vi "get git version.vi"(8 "error in":errorcluster) -> (0 "error out":errorcluster, 2 "hashcode":string, 3 "path to current head":path)   [LabVIEW 2013]
uses:
  <vilib>/regexp/Match Regular Expression.xnode
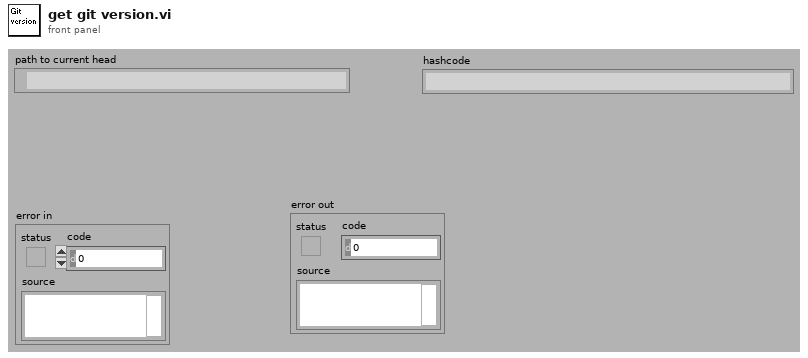
[diagram p1: front panel]
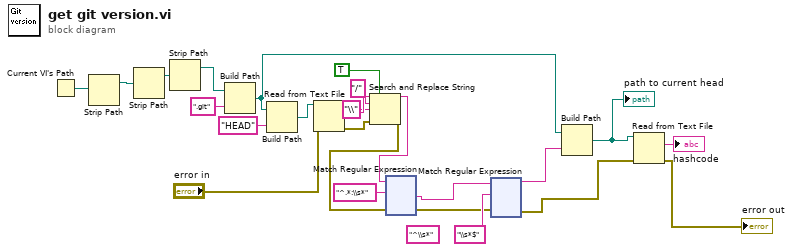
[diagram p0: block diagram]
diagram:
  (unwired) "^\\s*" ("regular expression")
  n1 = Current VI's Path() -> (path=w25:path)
  n2 = Strip Path(path=w25) -> (stripped path=w24:path)  [unwired: 1 out]
  n3 = Strip Path(path=w24) -> (stripped path=w23:path)  [unwired: 1 out]
  n4 = Strip Path(path=w23) -> (stripped path=w19:path)  [unwired: 1 out]
  n5 = Build Path(base path=w19, name or relative path=".git") -> (appended path=w10:path)
  n6 = Build Path(base path=w10, name or relative path="HEAD") -> (appended path=w20:path)
  n7 = Read from Text File(file (use dialog)=w20, error in="error in") -> (text=w18:string, error out=w5:errorcluster)  [unwired: 2 in, 2 out]
  n8 = Search and Replace String(replace all?=TRUE ("replace all? (F)"), input string=w18, search string="/", replace string="\\" ("replace string (\"\")"), error in=w5) -> (result string=w13:string, error out=w4:errorcluster)  [unwired: 3 in, 2 out]
  n9 = xnode "Match Regular Expression"("input string"=w13, "regular expression"="^.*:\\s*", "error in"=w4) -> ("after match"=w9:string, "error out"=w3:errorcluster)  [unwired: 3 in, 3 out]
  n10 = xnode "Match Regular Expression"("input string"=w9, "regular expression"="\\s*$", "error in"=w3) -> ("before match"=w11:string, "error out"=w2:errorcluster)  [unwired: 3 in, 3 out]
  n11 = Build Path(base path=w10, name or relative path=w11) -> (appended path=w8:path)
  "path to current head" <- w8
  n12 = Read from Text File(file (use dialog)=w8, error in=w2) -> (text=→"hashcode":string, error out=→"error out":errorcluster)  [unwired: 2 in, 2 out]
